vi "Write Value Defaults.vi"(9 "Value2":T1, 10 "Value1":T1, 11 "Effect Interface in":refnum<class "Effect Interface.lvclass">) -> (3 "Effect Interface out":refnum<class "Effect Interface.lvclass">)   [LabVIEW 2019, in "Effect Interface.lvlib" / "Effect Interface.lvclass"]
uses:
  Effect Interface.lvclass
  Libraries/Audio Processing/Value Cluster.ctl
  Libraries/Audio Processing/Value Properties.ctl
  Effect Interface.lvclass/Effect Interface.ctl
  Libraries/Audio Processing/Audio Processing.lvlib
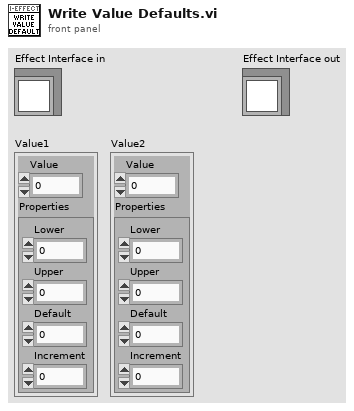
[diagram p1: front panel]
types:
  T1 = typedef "Audio Processing.lvlib/Value Cluster.ctl" = cluster{"Value":dbl, "Properties":T2}
  T2 = typedef "Audio Processing.lvlib/Value Properties.ctl" = cluster{"Lower":dbl, "Upper":dbl, "Default":dbl, "Increment":dbl}
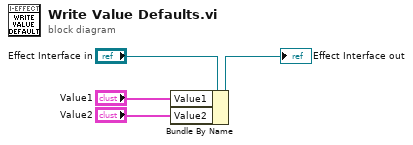
[diagram p0: block diagram]
diagram:
  n1 = Bundle By Name(cluster="Effect Interface in", "Value1"="Value1", "Value2"="Value2") -> (→"Effect Interface out":refnum<class "Effect Interface.lvclass">)
